vi "Analog Write Single.vi"(8 "error in (no error)":errorcluster, 9 "Analog Data":dbl, 10 "Channel Index":i32, 11 "Analog Writer in":refnum<class "Analog Writer.lvclass">) -> (0 "error out":errorcluster, 3 "Analog Writer out":refnum<class "Analog Writer.lvclass">)   [LabVIEW 2024, in "DAQmx Actor.lvlib" / "Analog Writer.lvclass"]
uses:
  Analog Writer.lvclass
  <vilib>/DAQmx/miscellaneous.llb/DAQmx Fill In Error Info.vi
  Analog Writer.lvclass/Analog Writer.ctl
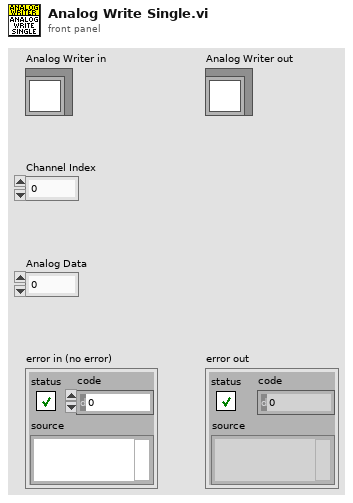
[diagram p1: front panel]
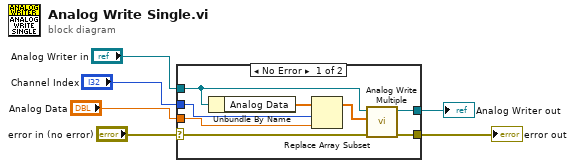
[diagram p0: block diagram]
diagram:
  n1 = case shown="No Error" "error in (no error)" {
    selector: "error in (no error)" -> [w7 w16]
    tunnel: [w8 w16] -> w5
    tunnel: [w9 w15] -> w3
    tunnel: "Analog Writer in" -> [w11 w15]
    tunnel: "Analog Data" -> [w12 _]
    tunnel: "Channel Index" -> [w14 _]
    frame No Error {
      n2 = Unbundle By Name(w11) -> ("Analog Data"=w13:dbl[])
      n3 = Replace Array Subset(array=w13, new element=w12, index=w14) -> (w10:dbl[])
      n4 = call-dynamic "Analog Write Multiple.vi"("error in (no error)"=w7, "Analog Data"=w10, "Analog Writer in"=w11) -> ("error out"=w8:errorcluster, "Analog Writer out"=w9:refnum<class "Analog Writer.lvclass">)  [unwired: 7 in]
    }
    frame Error {
    }
  }
  "error out" <- w5
  "Analog Writer out" <- w3
